vi "update.vi"(8 "error in (no error)":errorcluster, 11 "FPGAWrapperMH120124FrameScan_PXI7813R in":refnum<class "FPGAWrapperMH120124FrameScan_PXI7813R.lvclass">) -> (0 "error out":errorcluster, 3 "FPGAWrapperMH120124FrameScan_PXI7813R out":refnum<class "FPGAWrapperMH120124FrameScan_PXI7813R.lvclass">)   [LabVIEW 2010, in "FPGAWrapperMH120124FrameScan_PXI7813R.lvclass"]
uses:
  FPGAWrapperMH120124FrameScan_PXI7813R.lvclass
  grabber/command_enum.ctl
  FPGAWrapperMH120124FrameScan_PXI7813R.lvclass/FPGAWrapperMH120124FrameScan_PXI7813R.ctl
  class_data.vi
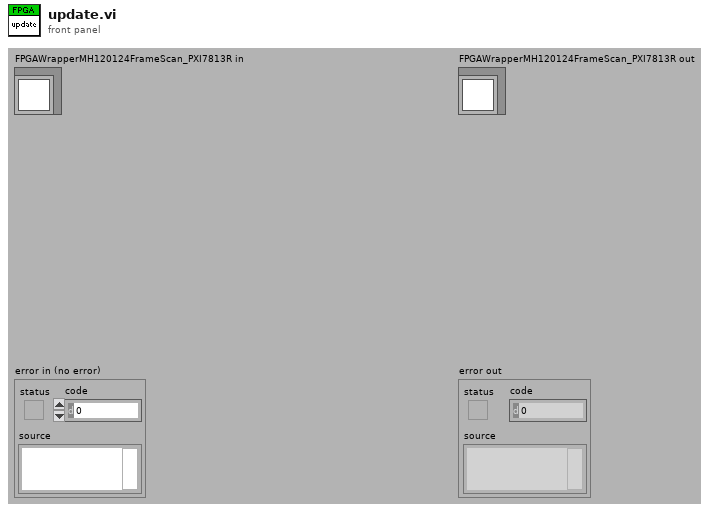
[diagram p1: front panel]
types:
  T1 = typedef "command_enum.ctl" = enum8{"NULL", "update", "start", "stop", "reset", "shut-down"}
  T2 = typedef "settings_cluster_framescan.ctl" = cluster{"number of pixels":i32, "iterations per pixel":i32, "maximum bit-depth":i8, "AOD center freq. (Hz)":dbl, "AOD bandwidth freq. (Hz)":dbl, "AOD amplitude":dbl, "pixel dwell time":dbl, "AOD equilibration time":dbl, "x resolution":i32, "y resolution":i32, "z angle (rotation angle, phi)":dbl, "x angle (tilting angle, phi)":dbl, "zoom":dbl, "pixel values cluster":T3, "offset (Hz)":dbl[], "DDS board initialization parameters":T4, "gates":T5[]}
  T3 = typedef "channels_cluster.ctl" = cluster{"channel 0":u32, "channel 1":u32, "channel 2":u32, "channel 3":u32}
  T4 = typedef "DDS_board_init_cluster.ctl" = cluster{"Bypass PLL":bool, "PLL Range":bool, "Update Clock":bool, "Triangle ":bool, "SDO Active":bool, "LSB First":bool, "OSK Int":bool, "Output Shaped Keying Enable":bool, "Bypass Sinc":bool, "Digital Part":bool, "OutPut DAC":bool, "Control DAC":bool, "Comparator":bool, "Modus":u8, "Multiplier Value":u8}
  T5 = typedef "gate_cluster.ctl" = cluster{"index":i32, "parameters":T6}
  T6 = typedef "gate_parameters_cluster.ctl" = cluster{"offset":i64, "pulsing":i64, "not pulsing":i64, "cycles per pulse":i64, "repetitions":i64}
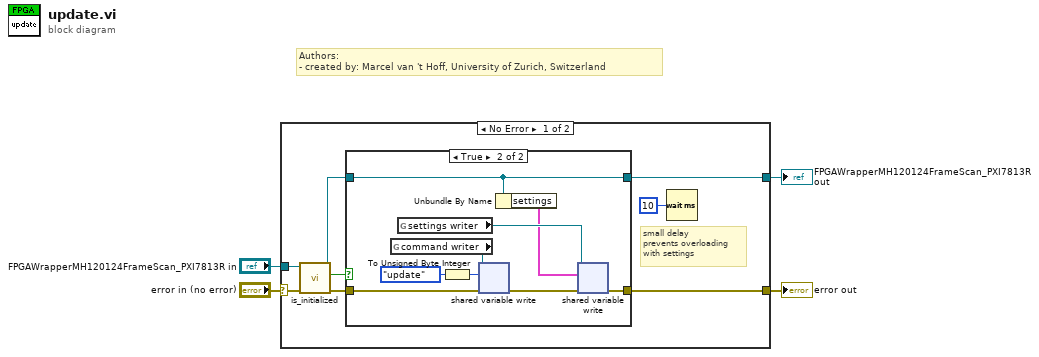
[diagram p0: block diagram]
diagram:
  # "Authors: \n- created by: Marcel van 't Hoff, University of Zurich, Switzerland"
  n1 = case shown="No Error" "error in (no error)" {
    selector: "error in (no error)" -> [w10 w25]
    tunnel: [w12 w25] -> w3
    tunnel: [w6 w24] -> w1
    tunnel: "FPGAWrapperMH120124FrameScan_PXI7813R in" -> [w11 w24]
    frame No Error {
      # "small delay\nprevents overloading\nwith settings"
      n2 = call-dynamic "is_initialized.vi"("error in (no error)"=w10, "FPGAWrapperMH120124FrameScan_PXI7813R in"=w11) -> ("error out"=w9:errorcluster, "is initialized?"=w8:bool, "FPGAWrapperMH120124FrameScan_PXI7813R out"=w7:refnum<class "FPGAWrapperMH120124FrameScan_PXI7813R.lvclass">)  [unwired: 7 in]
      n3 = case shown="True" w8 {
        tunnel: [w13 w17] -> w12
        tunnel: w7 -> [w14 w15]
        tunnel: w9 -> [w13 w16]
        tunnel: [w14 w15] -> w6
        frame False {
        }
        frame True {
          n4 = global read "class_data.vi" "command writer"() -> (w21:refnum<k21>)
          n5 = global read "class_data.vi" "settings writer"() -> (w19:refnum<k21>)
          n6 = To Unsigned Byte Integer(number=command_enum."update" ("command")) -> (unsigned 8bit integer=w23:u8)
          n7 = shared-variable-write(w21, w16, w23) -> (w20:errorcluster)  [unwired: 1 in, 2 out]
          n8 = Unbundle By Name(w15) -> ("settings"=w18:T2)
          n9 = shared-variable-write(w19, w20, w18) -> (w17:errorcluster)  [unwired: 1 in, 2 out]
        }
      }
      n10 = Wait (ms)(milliseconds to wait=u32 10) -> ()  [unwired: 1 out]
    }
    frame Error {
    }
  }
  "error out" <- w3
  "FPGAWrapperMH120124FrameScan_PXI7813R out" <- w1
